vi "Calculate Plot Range.vi"(8 "error in (no error)":errorcluster, 10 "2D Error Bar Datatype.lvclass in":refnum<class "2D Error Bar Datatype.lvclass">, 11 "Plot Representation In":T1) -> (0 "error out":errorcluster, 2 "2D Error Bar Datatype.lvclass out":refnum<class "2D Error Bar Datatype.lvclass">, 3 "Plot Representation Out":T1)   [LabVIEW 2020, in "2D Error Bar Datatype.lvclass"]
uses:
  <vilib>/Math Plots/2D Math Plots/2D Error Bar/2D Error Bar Datatype/2D Error Bar Datatype.lvclass
  <vilib>/Math Plots/2D Math Plots/2D Plot/2D Plot/Typedef/Plot Representation.ctl
  <vilib>/Math Plots/2D Math Plots/2D Plot/2D Plot/Typedef/Range Cluster.ctl
  <vilib>/Math Plots/2D Math Plots/2D Plot/2D Plot/2D Plot.lvclass
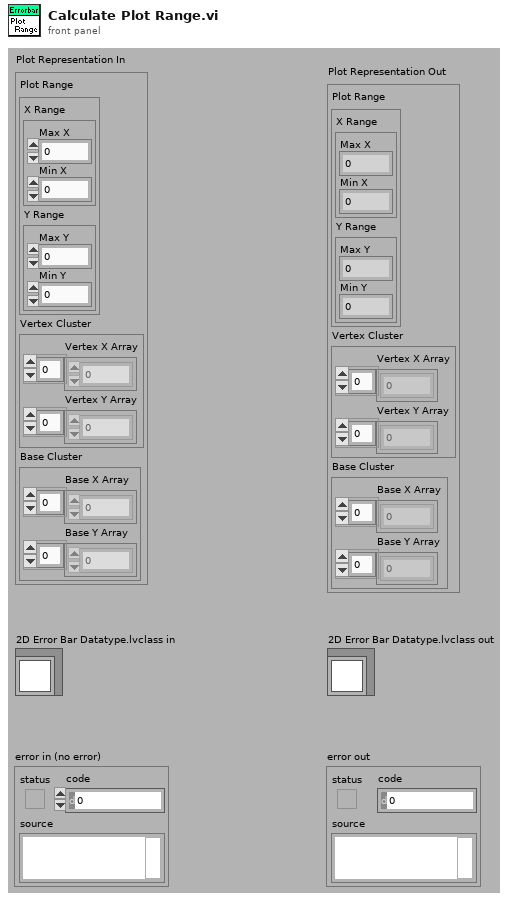
[diagram p1: front panel]
types:
  T1 = typedef "2D Plot.lvclass/Plot Representation.ctl" = cluster{"Plot Range":T2, "Vertex Cluster":cluster{"Vertex X Array":dbl[], "Vertex Y Array":dbl[]}, "Base Cluster":cluster{"Base X Array":dbl[], "Base Y Array":dbl[]}}
  T2 = typedef "2D Plot.lvclass/Range Cluster.ctl" = cluster{"X Range":cluster{"Max X":dbl, "Min X":dbl}, "Y Range":cluster{"Max Y":dbl, "Min Y":dbl}}
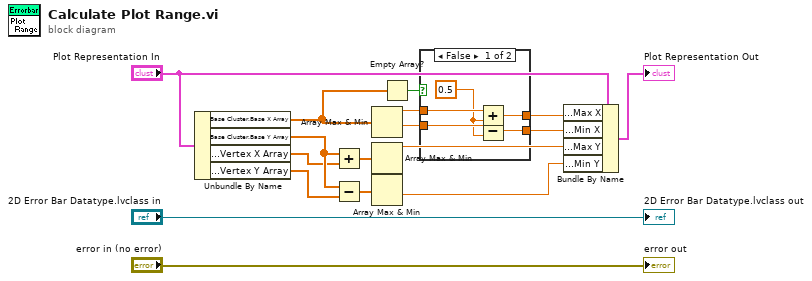
[diagram p0: block diagram]
diagram:
  n1 = Unbundle By Name("Plot Representation In") -> ("Base Cluster.Base X Array"=w2:dbl[], "Base Cluster.Base Y Array"=w11:dbl[], "Vertex Cluster.Vertex X Array"=w8:dbl[], "Vertex Cluster.Vertex Y Array"=w7:dbl[])
  n2 = Add(x=w11, y=w8) -> (x+y=w13:dbl[])
  n3 = Subtract(x=w11, y=w7) -> (x-y=w12:dbl[])
  n4 = Array Max & Min(array=w2) -> (max value=w6:dbl, min value=w4:dbl)  [unwired: 2 out]
  n5 = Array Max & Min(array=w13) -> (max value=w10:dbl)  [unwired: 3 out]
  n6 = Array Max & Min(array=w12) -> (min value=w9:dbl)  [unwired: 3 out]
  n7 = Empty Array?(array=w2) -> (empty?=w1:bool)
  n8 = case shown="False" w1 {
    tunnel: w6 -> [w22 w24]
    tunnel: [w21 w24] -> w5
    tunnel: w4 -> [w20 w23]
    tunnel: [w19 w23] -> w3
    frame False {
      w18 = 0.5 ("x")
      n9 = Add(x=w22, y=w18) -> (x+y=w21:dbl)
      n10 = Subtract(x=w20, y=w18) -> (x-y=w19:dbl)
    }
    frame True {
    }
  }
  n11 = Bundle By Name(cluster="Plot Representation In", "Plot Range.X Range.Max X"=w5, "Plot Range.X Range.Min X"=w3, "Plot Range.Y Range.Max Y"=w10, "Plot Range.Y Range.Min Y"=w9) -> (→"Plot Representation Out":T1)
  "2D Error Bar Datatype.lvclass out" <- "2D Error Bar Datatype.lvclass in"
  "error out" <- "error in (no error)"
